vi "subvi.vi"() -> ()   [LabVIEW 2021]
panel:
  in  "stop":bool
  out "C":dbl
  in  "Numeric":dbl
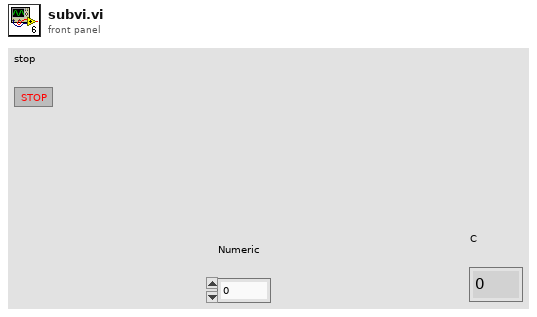
[diagram p1: front panel]
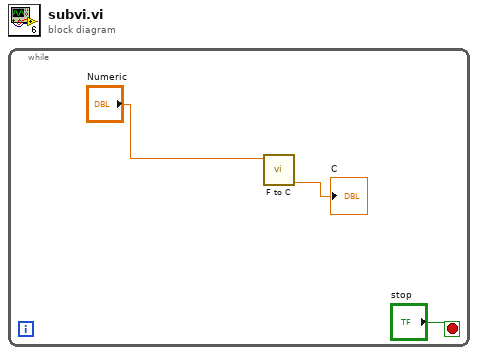
[diagram p0: block diagram]
diagram:
  n1 = while {
    stop <- "stop" stop-if-true
    n2 = call "F to C.vi"("F"="Numeric") -> ("C"=→"C":dbl)  [unwired: 10 in]
  }
